vi "Log Message.vi"(8 "error in (no error)":errorcluster, 10 "message":string, 11 "WebSocket Logger in":refnum<class "WebSocket Logger.lvclass">) -> (0 "error out":errorcluster, 3 "WebSocket Logger out":refnum<class "WebSocket Logger.lvclass">)   [LabVIEW 2019, in "WebSocket Server Toolkit.lvlib" / "WebSocket Logger.lvclass"]
uses:
  WebSocket Logger.lvclass
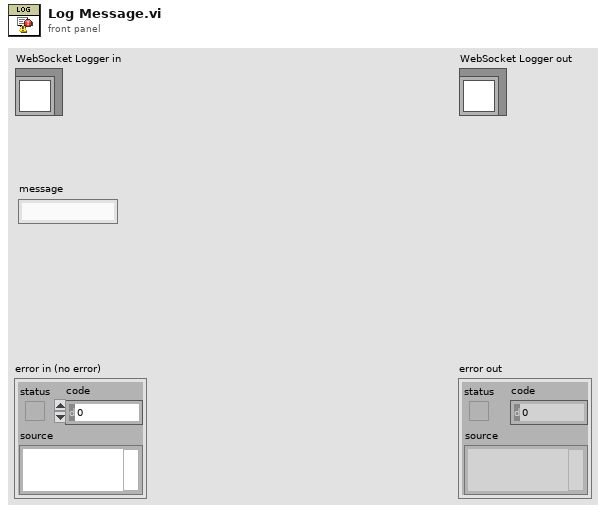
[diagram p1: front panel]
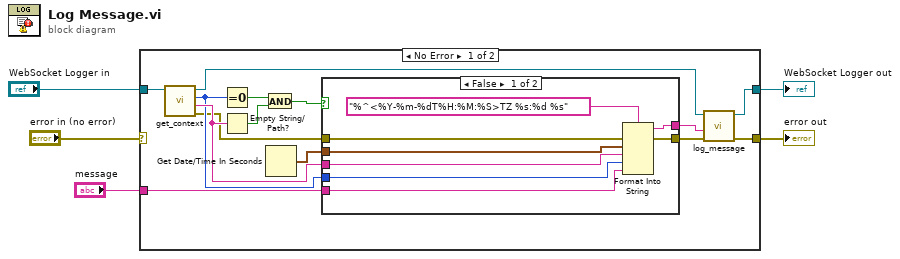
[diagram p0: block diagram]
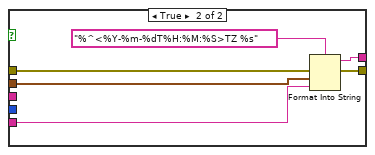
[diagram p2: hidden frame]
diagram:
  n1 = case shown="No Error" "error in (no error)" {
    selector: "error in (no error)" -> [_ w35]
    tunnel: [w6 w35] -> w4
    tunnel: [w17 w34] -> w2
    tunnel: "WebSocket Logger in" -> [w19 w34]
    tunnel: "message" -> [w12 _]
    frame No Error {
      n2 = call-dynamic "get_context.vi"("WebSocket Logger in"=w19) -> ("error out"=w8:errorcluster, "remote address"=w11:string, "remote port"=w10:u16, "WebSocket Logger out"=w18:refnum<class "WebSocket Logger.lvclass">)  [unwired: 7 in]
      n3 = Equal To 0?(x=w10) -> (x = 0?=w16:bool)
      n4 = Empty String/Path?(string/path=w11) -> (empty?=w15:bool)
      n5 = And(x=w16, y=w15) -> (x .and. y?=w14:bool)
      n6 = Get Date/Time In Seconds() -> (seconds since 1Jan1904=w13:timestamp)
      n7 = case shown="False" w14 {
        tunnel: w13 -> [w26 w32]
        tunnel: w12 -> [w25 w31]
        tunnel: w11 -> [w24 _]
        tunnel: w10 -> [w23 _]
        tunnel: [w22 w30] -> w9
        tunnel: w8 -> [w20 w29]
        tunnel: [w21 w28] -> w7
        frame False {
          n8 = Format Into String(format string="%^<%Y-%m-%dT%H:%M:%S>TZ %s:%d %s", error in=w20, w26, w24, w23, w25) -> (resulting string=w22:string, error out=w21:errorcluster)  [unwired: 1 in]
        }
        frame True {
          n9 = Format Into String(format string="%^<%Y-%m-%dT%H:%M:%S>TZ %s", error in=w29, w32, w31) -> (resulting string=w30:string, error out=w28:errorcluster)  [unwired: 1 in]
        }
      }
      n10 = call-dynamic "log_message.vi"("error in (no error)"=w7, "message"=w9, "Logger in"=w18) -> ("error out"=w6:errorcluster, "Logger out"=w17:refnum<class "WebSocket Logger.lvclass">)  [unwired: 7 in]
    }
    frame Error {
    }
  }
  "error out" <- w4
  "WebSocket Logger out" <- w2
